vi "Initialize.vi"(0 "Application in":refnum<class "Application.lvclass">, 5 "error in (no error)":errorcluster) -> (14 "Application out":refnum<class "Application.lvclass">, 19 "error out":errorcluster)   [LabVIEW 2019, in "Application.lvclass"]
uses:
  Application.lvclass
  Application.lvclass/Application.ctl
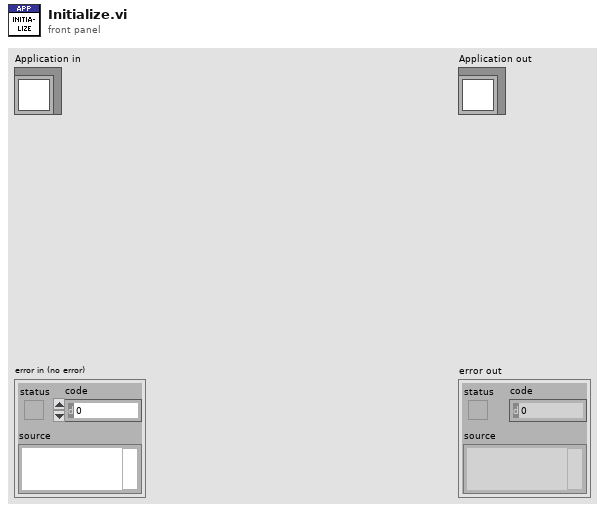
[diagram p1: front panel]
types:
  T1 = typedef "NI_LVConfig.lvlib/Config Data RefNum.ctl" = refnum<k1>
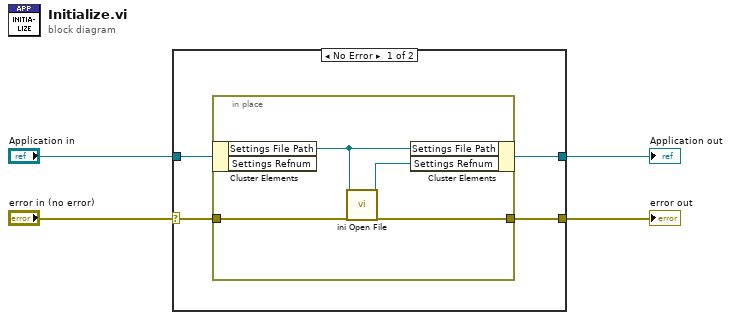
[diagram p0: block diagram]
diagram:
  n1 = case shown="No Error" "error in (no error)" {
    selector: "error in (no error)" -> [w6 w14]
    tunnel: [w5 w14] -> w3
    tunnel: [w7 w13] -> w1
    tunnel: "Application in" -> [w8 w13]
    frame No Error {
      n2 = in-place {
        in-place-border: w6 -> [w10]
        in-place-border: [w9] -> w5
        n3 = in-place-cluster #1(w8) -> ("Settings File Path"=w12:path)  [unwired: 1 out]
        n4 = call "ini Open File.vi"("ini File"=w12, "Error In"=w10) -> ("ini Refnum"=w11:T1, "Error Out"=w9:errorcluster)  [unwired: 16 in]
        n5 = in-place-cluster #1("Settings File Path"=w12, "Settings Refnum"=w11) -> (w7:refnum<class "Application.lvclass">)
      }
    }
    frame Error {
    }
  }
  "error out" <- w3
  "Application out" <- w1
